vi "Test TCP Socket.vi"() -> ()   [LabVIEW 2023]
panel:
  out "data out 2":string
  out "value":T1
  in  "Cluster":T1
  out "data string":string
  out "concatenated string":string
  out "data out":string
  out "error out":errorcluster
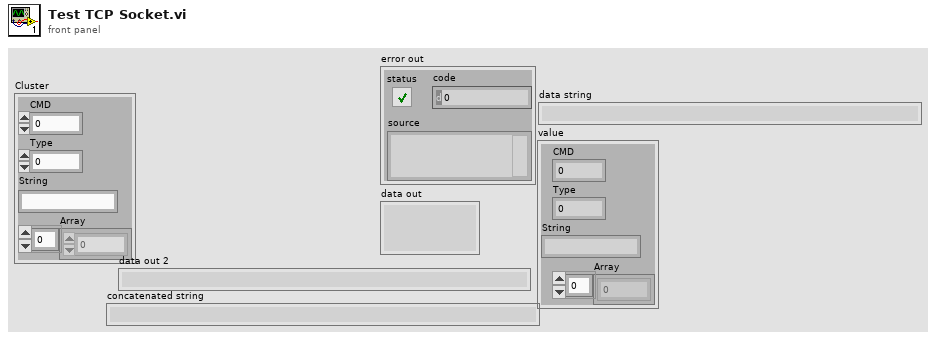
[diagram p1: front panel]
types:
  T1 = cluster{"CMD":u8, "Type":u8, "String":string, "Array":u8[]}
  T2 = enum16{"big-endian, network order", "native, host order", "little-endian"}
  T3 = enum16{"Standard", "Buffered", "CRLF", "Immediate"}
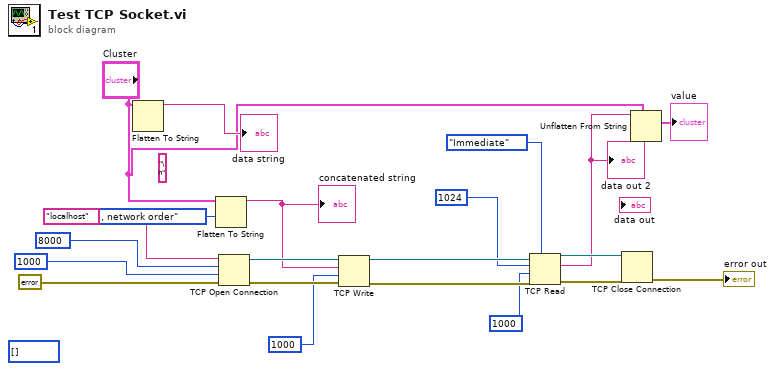
[diagram p0: block diagram]
diagram:
  (unwired) u8[] []
  (unwired) "\n"
  n1 = Flatten To String(anything="Cluster") -> (data string=→"data string":string)  [unwired: 3 in, 2 out]
  n2 = Flatten To String(anything="Cluster", byte order (0:big-endian, network order)=T2."big-endian, network order") -> (data string=w1:string)  [unwired: 2 in, 2 out]
  "concatenated string" <- w1
  n3 = TCP Open Connection(address="localhost", remote port or service name=u16 8000, timeout ms (60000)=1000, error in (no error)=errorcluster {"status"=FALSE, "code"=0, "source"=""}) -> (connection ID=w17:refnum<k5>, error out=w16:errorcluster)  [unwired: 1 in]
  n4 = TCP Write(connection ID=w17, data in=w1, error in (no error)=w16, 9:1000 ("timeout ms (25000)")) -> (connection ID out=w14:refnum<k5>, error out=w13:errorcluster)  [unwired: 1 out]
  n5 = TCP Read(connection ID=w14, bytes to read=1024, error in (no error)=w13, 7:T3."Immediate" ("mode (standard)"), 9:1000 ("timeout ms (25000)")) -> (connection ID out=w9:refnum<k5>, data out=w5:string, error out=w8:errorcluster)
  "data out 2" <- w5
  n6 = TCP Close Connection(connection ID=w9, error in (no error)=w8) -> (error out=→"error out":errorcluster)  [unwired: 1 in, 1 out]
  n7 = Unflatten From String(type="Cluster", binary string=w5) -> (value=→"value":T1)  [unwired: 3 in, 2 out]
